vi "AppInfo.vi"() -> ()   [LabVIEW 2017]
panel:
  in  "OK":bool
  out "HowTo":string
  # "Informações"
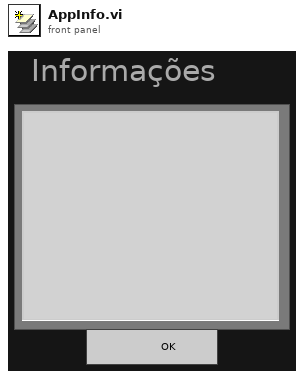
[diagram p1: front panel]
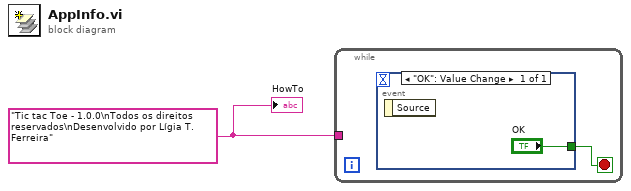
[diagram p0: block diagram]
diagram:
  w1 = "Tic tac Toe - 1.0.0\nTodos os direitos reservados\nDesenvolvido por Lígia T. Ferreira"
  n1 = while {
    tunnel: w1 -> [_]
    stop <- w2 stop-if-true
    n2 = event shown="[0] \"OK\": Value Change" {
      selector: _ -> [_]
      dyn-events: _ -> [_]
      timeout: _ -> [_]
      tunnel: ["OK"] -> w2
      event "OK": Value Change {
        n3 = event-data() -> ()  [unwired: 1 in, 1 out]
      }
    }
  }
  "HowTo" <- w1
